vi "Swap Limit Switches.vi"(8 "error in (no error)":errorcluster, 9 "Swap":bool, 10 "Index":i32, 11 "Visa Array in":refnum<visa-resource-name>[](array[refnum])) -> (0 "error out":errorcluster, 3 "Visa Array out":refnum<visa-resource-name>[](array[refnum]))   [LabVIEW 2010, in "SignalWriterMH110203USBStepperMotor.lvclass"]
uses:
  SignalWriterMH110203USBStepperMotor.lvclass
  class_data.vi
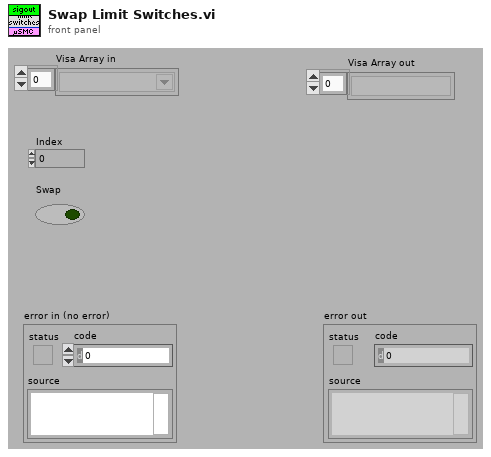
[diagram p1: front panel]
types:
  T1 = typedef "SignalWriterMH110203USBStepperMotor.lvclass/Mode Control (uSMC).ctl" = cluster{"Turn Buttons Off":bool, "Reduce Current":bool, "Power Off and Make a Whole Step":bool, "Emergency Power Off":bool, "Limit Switch 1 True State":bool, "Limit Switch 2 True State":bool, "Rotary Transducer TRUE State":bool, "Swap Limit Switches":bool, "Limit Switch 1 Operation Enabled":bool, "Limit Switch 2 Operation Enabled":bool, "Rotary Transducer Operation Enabled":bool, "Rotary Transducer Operation Select":bool, "Button 1 True State":bool, "Button 2 True State":bool, "Swap Buttons":bool, "Reset Rotary Transducer Check Positions":bool, "Output Syncronization Enabled":bool, "Reset Output Sync Count":bool, "Sync Operation":bool, "Sync Count":u32, "Power":bool, "Invert Sync Polarity":bool, "Use Encoder":bool, "Invert Encoder Direction":bool, "Reset Encoder To 0":bool, "Reset SM Enc Pos to Enc Pos":bool}
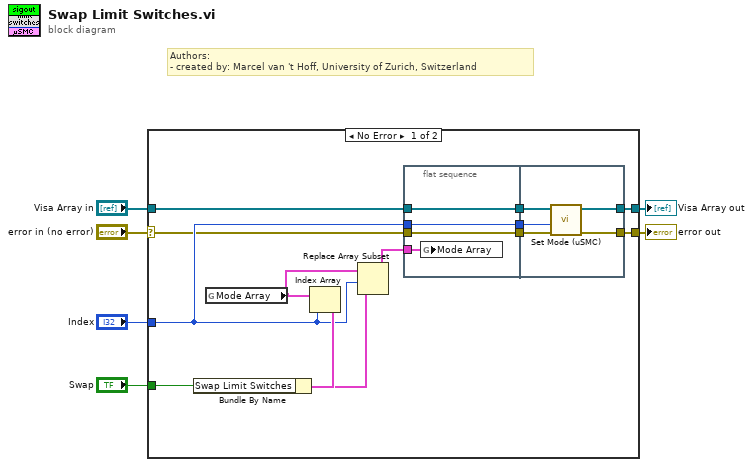
[diagram p0: block diagram]
diagram:
  # "Authors: \n- created by: Marcel van 't Hoff, University of Zurich, Switzerland"
  n1 = case shown="No Error" "error in (no error)" {
    selector: "error in (no error)" -> [w7 w30]
    tunnel: "Visa Array in" -> [w16 w29]
    tunnel: [w15 w29] -> w5
    tunnel: [w14 w30] -> w4
    tunnel: "Swap" -> [w12 _]
    tunnel: "Index" -> [w9 _]
    frame No Error {
      n2 = global read "class_data.vi" "Mode Array"() -> (w10:T1[])
      n3 = Index Array(array=w10, index=w9) -> (element=w13:T1)
      n4 = Bundle By Name(cluster=w13, "Swap Limit Switches"=w12) -> (w11:T1)
      n5 = Replace Array Subset(array=w10, new element=w11, index=w9) -> (w8:T1[])
      n6 = flat-sequence {
        tunnel: w9 -> [w21]
        tunnel: w7 -> [w22]
        tunnel: w16 -> [w23]
        tunnel: [w23] -> w19
        tunnel: [w22] -> w18
        tunnel: [w21] -> w17
        tunnel: w8 -> [w20]
        tunnel: [w27] -> w15
        tunnel: [w25] -> w14
        tunnel: w19 -> [w28]
        tunnel: w18 -> [w26]
        tunnel: w17 -> [w24]
        frame #0 {
          n7 = global write "class_data.vi" "Mode Array"(w20) -> ()
        }
        frame #1 {
          n8 = call "Set Mode (uSMC).vi"("error in (no error)"=w26, "Index"=w24, "Visa Array in"=w28) -> ("error out"=w25:errorcluster, "Visa Array out"=w27:refnum<visa-resource-name>[])  [unwired: 7 in]
        }
      }
    }
    frame Error {
    }
  }
  "Visa Array out" <- w5
  "error out" <- w4
